vi "Layout.vi"(8 "error in (no error)":errorcluster, 11 "FSM in":refnum<class "FSM.Node.lvclass">) -> (0 "error out":errorcluster, 3 "FSM out":refnum<class "FSM.Node.lvclass">)   [LabVIEW 2015, in "FSM.Node.lvclass"]
uses:
  FSM.Node.lvclass
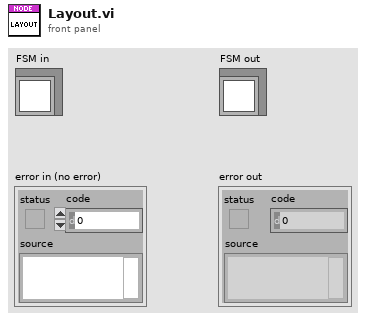
[diagram p1: front panel]
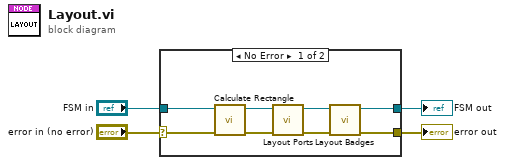
[diagram p0: block diagram]
diagram:
  n1 = case shown="No Error" "error in (no error)" {
    selector: "error in (no error)" -> [w11 w14]
    tunnel: [w5 w14] -> w3
    tunnel: [w7 w13] -> w1
    tunnel: "FSM in" -> [w12 w13]
    frame No Error {
      n2 = call "Calculate Rectangle.vi"("error in (no error)"=w11, "FSM.Node in"=w12) -> ("error out"=w9:errorcluster, "FSM.Node out"=w10:refnum<class "FSM.Node.lvclass">)  [unwired: 8 in]
      n3 = call "Layout Ports.vi"("error in (no error)"=w9, "Node in"=w10) -> ("error out"=w6:errorcluster, "Node out"=w8:refnum<class "FSM.Node.lvclass">)  [unwired: 8 in]
      n4 = call "Layout Badges.vi"("error in (no error)"=w6, "Node in"=w8) -> ("error out"=w5:errorcluster, "Node out"=w7:refnum<class "FSM.Node.lvclass">)  [unwired: 8 in]
    }
    frame Error {
    }
  }
  "error out" <- w3
  "FSM out" <- w1
